vi "test_reqrep.vi"() -> ()   [LabVIEW 2019]
uses:
  socket_type.ctl
  error_type.ctl
  zmq_socket.lvclass
  zmq_context.lvclass
  zeromq.lvlib
panel:
  out "terminated":bool
  out "poll recv":bool
  out "send multi":bool
  out "recv multi":bool
  out "error out":errorcluster
  out "timeout":bool
  out "zmq ver":string
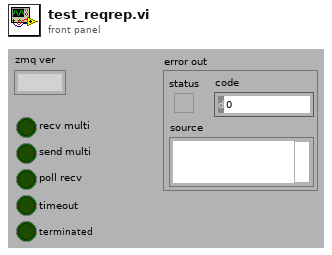
[diagram p1: front panel]
types:
  T1 = typedef "zeromq.lvlib/error_type.ctl" = enum16{"No Error", "EUNKNOWN", "ENOTSUP", "EPROTONOSUPPORT", "ENOBUFS", "ENETDOWN", "EADDRINUSE", "EADDRNOTAVAIL", "ECONNREFUSED", "EINPROGRESS", "ENOTSOCK", "EMSGSIZE", "EAFNOSUPPORT", "ENETUNREACH", "ECONNABORT", "ECONNRESET", "ENOTCONN", "ETIMEDOUT", "EHOSTUNREACH", "ENETRESET", "EBUSY", "EINVAL", "ENODEV", "EFAULT", "EINTR", "ENOENT", "ENOMEM", "EAGAIN", "EMFILE", "EFSM", "ENOCOMPATPROTO", "ETERM", "EMTHREAD", "Invalid"}
  T2 = typedef "zeromq.lvlib/socket_type.ctl" = enum8{"ZMQ_PAIR", "ZMQ_PUB", "ZMQ_SUB", "ZMQ_REQ", "ZMQ_REP", "ZMQ_DEALER", "ZMQ_ROUTER", "ZMQ_PULL", "ZMQ_PUSH", "ZMQ_XPUB", "ZMQ_XSUB"}
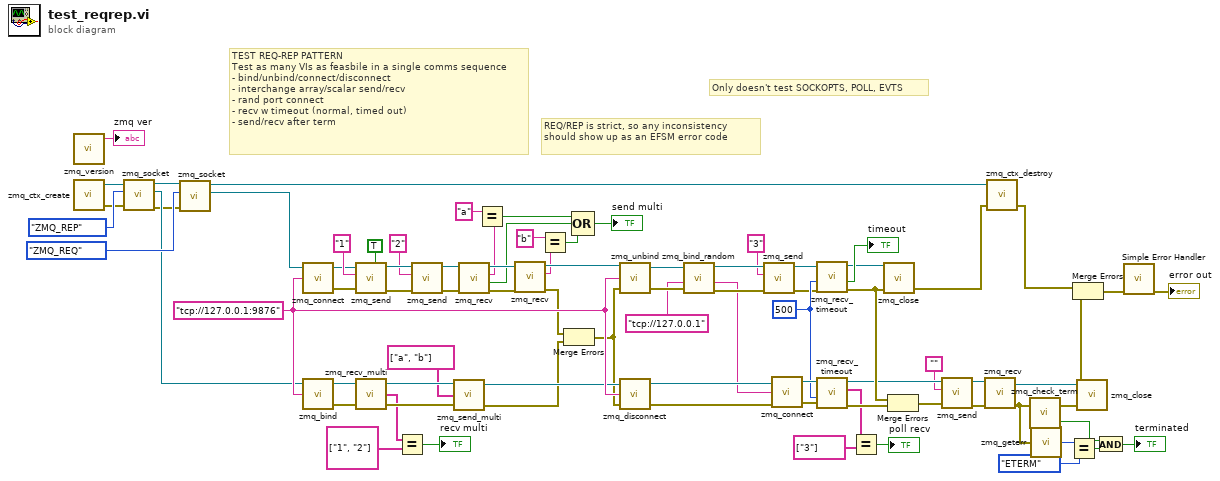
[diagram p0: block diagram]
diagram:
  w59 = u32 500 ("timeout (ms)")
  w75 = "tcp://127.0.0.1:9876"
  # "Only doesn't test SOCKOPTS, POLL, EVTS"
  # "TEST REQ-REP PATTERN\nTest as many VIs as feasbile in a single comms sequence\n- bind/unbind/connect/disconnect\n- interchange array/scalar send/recv\n- rand port connect\n- recv w timeout (normal, timed out)\n- send/recv after term"
  # "REQ/REP is strict, so any inconsistency should show up as an EFSM error code"
  n1 = call "zmq_version.vi"() -> ("version string"=→"zmq ver":string)  [unwired: 3 in, 2 out]
  n2 = call "zmq_ctx_create.vi"() -> ("error out"=w4:errorcluster, "context out"=w6:refnum<class "zmq_context.lvclass">)  [unwired: 4 in]
  n3 = call "zmq_socket.vi"("error in"=w4, "socket type"=socket_type."ZMQ_REP", "context in"=w6) -> ("error out"=w3:errorcluster, "socket out"=w8:refnum<class "zmq_socket.lvclass">, "context out"=w7:refnum<class "zmq_context.lvclass">)  [unwired: 2 in]
  n4 = call "zmq_socket.vi"("error in"=w3, "socket type"=socket_type."ZMQ_REQ", "context in"=w7) -> ("socket out"=w9:refnum<class "zmq_socket.lvclass">, "context out"=w5:refnum<class "zmq_context.lvclass">)  [unwired: 2 in, 1 out]
  n5 = call "zmq_connect.vi"("endpoint"=w75, "socket in"=w9) -> ("error out"=w46:errorcluster, "socket out"=w47:refnum<class "zmq_socket.lvclass">)  [unwired: 2 in]
  n6 = call "zmq_bind.vi"("endpoint"=w75, "socket in"=w8) -> ("error out"=w48:errorcluster, "socket out"=w49:refnum<class "zmq_socket.lvclass">)  [unwired: 2 in]
  n7 = call "zmq_send.vi"("error in"=w46, "data"="1", "socket in"=w47, "more? (F)"=TRUE) -> ("error out"=w70:errorcluster, "socket out"=w79:refnum<class "zmq_socket.lvclass">)  [unwired: 3 in]
  n8 = call "zmq_recv_multi.vi"("error in"=w48, "socket in"=w49) -> ("error out"=w52:errorcluster, "parts"=w33:string[], "socket out"=w53:refnum<class "zmq_socket.lvclass">)  [unwired: 1 in]
  n9 = Equal?(x=w33, y=string[] ["1", "2"] ("12")) -> (x = y?=→"recv multi":bool)
  n10 = call "zmq_send.vi"("error in"=w70, "data"="2", "socket in"=w79) -> ("error out"=w55:errorcluster, "socket out"=w58:refnum<class "zmq_socket.lvclass">)  [unwired: 4 in]
  n11 = call "zmq_send_multi.vi"("error in"=w52, "parts"=string[] ["a", "b"], "socket in"=w53) -> ("error out"=w18:errorcluster, "socket out"=w50:refnum<class "zmq_socket.lvclass">)  [unwired: 1 in]
  n12 = call "zmq_recv.vi"("error in"=w55, "socket in"=w58) -> ("error out"=w54:errorcluster, "more?"=w25:bool, "data"=w30:string, "socket out"=w57:refnum<class "zmq_socket.lvclass">)  [unwired: 3 in, 1 out]
  n13 = Equal?(x="a" ("a"), y=w30) -> (x = y?=w27:bool)
  n14 = call "zmq_recv.vi"("error in"=w54, "socket in"=w57) -> ("error out"=w19:errorcluster, "data"=w29:string, "socket out"=w56:refnum<class "zmq_socket.lvclass">)  [unwired: 3 in, 2 out]
  n15 = Equal?(x="b" ("b"), y=w29) -> (x = y?=w26:bool)
  n16 = Merge Errors(w19, w18) -> (w17:errorcluster)
  n17 = Compound Arithmetic op=OR(w27, w25, w26) -> (→"send multi":bool)
  n18 = call "zmq_unbind.vi"("error in"=w17, "endpoint"=w75, "socket in"=w56) -> ("error out"=w69:errorcluster, "socket out"=w77:refnum<class "zmq_socket.lvclass">)  [unwired: 1 in]
  n19 = call "zmq_disconnect.vi"("error in"=w17, "endpoint"=w75, "socket in"=w50) -> ("error out"=w67:errorcluster, "socket out"=w74:refnum<class "zmq_socket.lvclass">)  [unwired: 1 in]
  n20 = call "zmq_bind_random.vi"("error in"=w69, "base"="tcp://127.0.0.1", "socket in"=w77) -> ("error out"=w68:errorcluster, "endpoint"=w1:string, "socket out"=w76:refnum<class "zmq_socket.lvclass">)  [unwired: 1 in, 1 out]
  n21 = call "zmq_send.vi"("error in"=w68, "data"="3", "socket in"=w76) -> ("error out"=w44:errorcluster, "socket out"=w45:refnum<class "zmq_socket.lvclass">)  [unwired: 4 in]
  n22 = call "zmq_connect.vi"("error in"=w67, "endpoint"=w1, "socket in"=w74) -> ("error out"=w66:errorcluster, "socket out"=w73:refnum<class "zmq_socket.lvclass">)  [unwired: 1 in]
  n23 = call "zmq_recv_timeout.vi"("error in"=w44, "timeout (ms)"=w59, "socket in"=w45) -> ("error out"=w42:errorcluster, "timeout?"=→"timeout":bool, "socket out"=w43:refnum<class "zmq_socket.lvclass">)  [unwired: 1 in, 1 out]
  n24 = call "zmq_recv_timeout.vi"("error in"=w66, "timeout (ms)"=w59, "socket in"=w73) -> ("error out"=w41:errorcluster, "parts"=w22:string[], "socket out"=w38:refnum<class "zmq_socket.lvclass">)  [unwired: 1 in, 1 out]
  n25 = Equal?(x=w22, y=string[] ["3"] ("3")) -> (x = y?=→"poll recv":bool)
  n26 = call "zmq_close.vi"("error in"=w42, "socket"=w43) -> ("error out"=w35:errorcluster)  [unwired: 3 in]
  n27 = Merge Errors(w42, w41) -> (w40:errorcluster)
  n28 = call "zmq_send.vi"("error in"=w40, "data"="", "socket in"=w38) -> ("error out"=w39:errorcluster, "socket out"=w37:refnum<class "zmq_socket.lvclass">)  [unwired: 4 in]
  n29 = call "zmq_recv.vi"("error in"=w39, "socket in"=w37) -> ("error out"=w16:errorcluster, "socket out"=w71:refnum<class "zmq_socket.lvclass">)  [unwired: 3 in, 3 out]
  n30 = call "zmq_ctx_destroy.vi"("error in"=w35, "context in"=w5) -> ("error out"=w65:errorcluster)  [unwired: 3 in]
  n31 = call "zmq_check_term.vi"("error in"=w16) -> ("term?"=w12:bool, "error out"=w72:errorcluster)  [unwired: 1 in]
  n32 = call "zmq_geterr.vi"("error in"=w16) -> ("type"=w15:T1)
  n33 = Equal?(x=w15, y=error_type."ETERM") -> (x = y?=w13:bool)
  n34 = call "zmq_close.vi"("error in"=w72, "socket"=w71) -> ("error out"=w64:errorcluster)  [unwired: 3 in]
  n35 = Merge Errors(w65, w64) -> (w20:errorcluster)
  n36 = And(x=w12, y=w13) -> (x .and. y?=→"terminated":bool)
  n37 = call <vilib>:"Simple Error Handler.vi"("error in (no error)"=w20) -> ("error out"=→"error out":errorcluster)  [unwired: 4 in, 4 out]
